vi "SP Determine Data Format From Limit Format.vi"(1 "Limit Format":T1) -> (0 "Format String":string)   [LabVIEW 2011]
uses:
  TypeDefs/SP Format.ctl
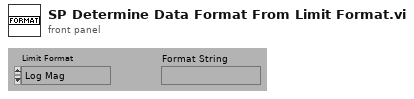
[diagram p1: front panel]
types:
  T1 = typedef "SP Format.ctl" = enum16{"Log Mag", "Lin Mag", "SWR", "Phase", "Expanded Phase", "Delay", "Insertion Loss", "Isolation", "Return Loss"}
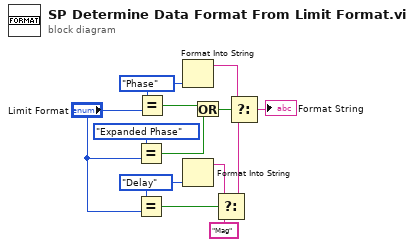
[diagram p0: block diagram]
diagram:
  w5 = SP_Format."Delay" ("x")
  w2 = SP_Format."Phase" ("x")
  n1 = Equal?(x=SP_Format."Expanded Phase", y="Limit Format") -> (x = y?=w12:bool)
  n2 = Equal?(x=w5, y="Limit Format") -> (x = y?=w4:bool)
  n3 = Equal?(x=w2, y="Limit Format") -> (x = y?=w13:bool)
  n4 = Format Into String(w2) -> (resulting string=w3:string)  [unwired: 3 in, 1 out]
  n5 = Format Into String(w5) -> (resulting string=w6:string)  [unwired: 3 in, 1 out]
  n6 = Or(x=w13, y=w12) -> (x .or. y?=w9:bool)
  n7 = Select(t=w6, s=w4, f="Mag") -> (s? t:f=w7:string)
  n8 = Select(t=w3, s=w9, f=w7) -> (s? t:f=→"Format String":string)
